vi "Kinesis-basic_program.vi"() -> ()   [LabVIEW 2014]
doc: "André Romero - 2017\nandretec@ifsc.usp.br"
panel:
  out "Numeric 2":i32
  out "GetPOS Y":dbl=10.0
  out "GetPOS X":dbl=10.0 format="%^#1_6e"
  in  "GO Move":bool
  out "Motor 2":bool
  out "Motor 1":bool
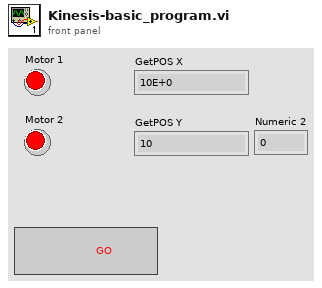
[diagram p1: front panel]
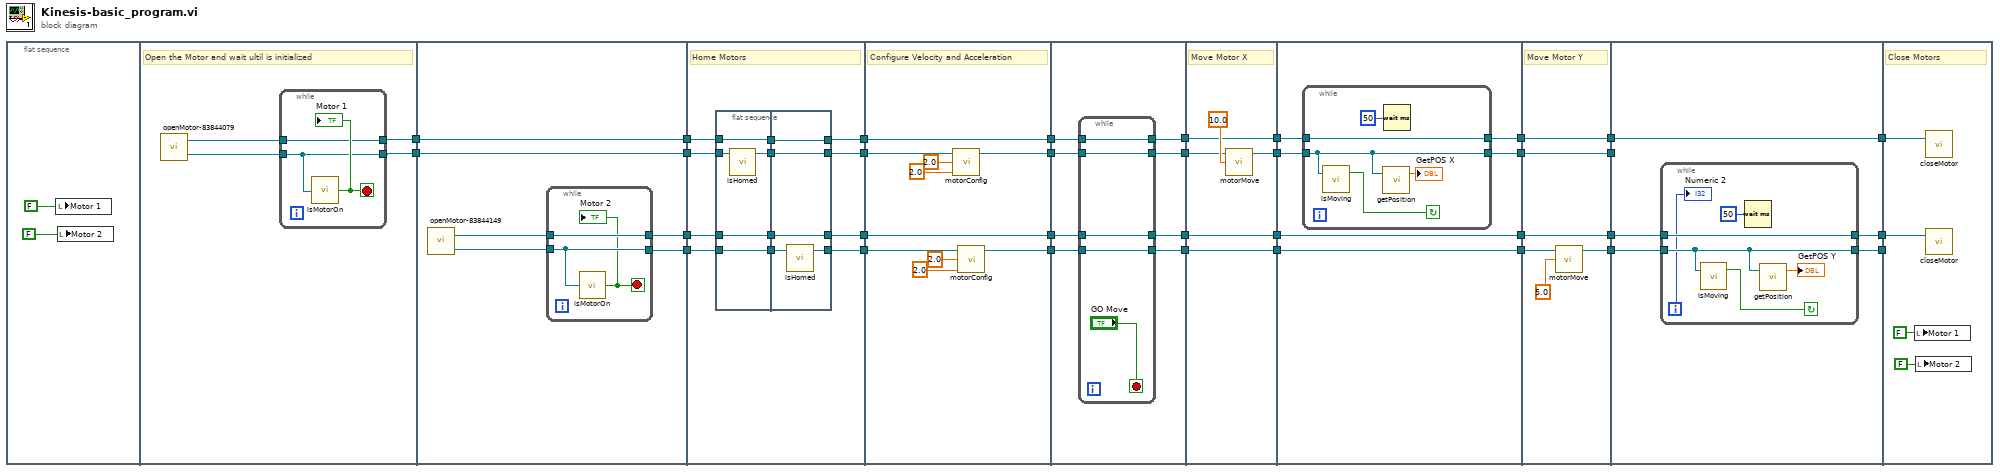
[diagram p0: block diagram]
diagram:
  n1 = flat-sequence {
    tunnel: [w39] -> w10
    tunnel: [w38] -> w8
    tunnel: w10 -> [w48]
    tunnel: [w48] -> w9
    tunnel: w8 -> [w47]
    tunnel: [w47] -> w7
    tunnel: [w46] -> w6
    tunnel: [w45] -> w5
    tunnel: w9 -> [w59]
    tunnel: w7 -> [w58]
    tunnel: [w61] -> w31
    tunnel: w6 -> [w60]
    tunnel: [w62] -> w29
    tunnel: w5 -> [w63]
    tunnel: [w55] -> w33
    tunnel: [w54] -> w27
    tunnel: w33 -> [w82]
    tunnel: [w82] -> w32
    tunnel: w31 -> [w83]
    tunnel: [w83] -> w30
    tunnel: w29 -> [w81]
    tunnel: [w78] -> w28
    tunnel: w27 -> [w74]
    tunnel: [w75] -> w26
    tunnel: w32 -> [w91]
    tunnel: [w90] -> w19
    tunnel: w30 -> [w87]
    tunnel: [w84] -> w22
    tunnel: w28 -> [w85]
    tunnel: [w86] -> w21
    tunnel: w26 -> [w88]
    tunnel: [w89] -> w20
    tunnel: w22 -> [w102]
    tunnel: [w102] -> w18
    tunnel: w21 -> [w97]
    tunnel: [w97] -> w17
    tunnel: w20 -> [w99]
    tunnel: [w98] -> w16
    tunnel: w19 -> [w100]
    tunnel: [w100] -> w15
    tunnel: w18 -> [w104]
    tunnel: [w104] -> w14
    tunnel: w17 -> [w103]
    tunnel: w16 -> [w105]
    tunnel: [w106] -> w13
    tunnel: w15 -> [w108]
    tunnel: [w107] -> w12
    tunnel: [w103] -> w11
    tunnel: w14 -> [w119]
    tunnel: [w119] -> w4
    tunnel: [w114] -> w3
    tunnel: w13 -> [w118]
    tunnel: [w118] -> w2
    tunnel: w12 -> [w117]
    tunnel: [w117] -> w1
    tunnel: w11 -> [w115]
    tunnel: w4 -> [w124]
    tunnel: [w123] -> w25
    tunnel: w3 -> [w120]
    tunnel: [w122] -> w24
    tunnel: w2 -> [_]
    tunnel: w1 -> [w121]
    tunnel: [w121] -> w23
    tunnel: w25 -> [w133]
    tunnel: w24 -> [_]
    tunnel: w23 -> [w134]
    frame #0 {
      n2 = local write "Motor 1"(FALSE ("isConnected")) -> ()
      n3 = local write "Motor 2"(FALSE ("isConnected 2")) -> ()
    }
    frame #1 {
      # "Open the Motor and wait ultil is initialized"
      n4 = call "openMotor-83844079.vi"() -> ("Device"=w37:refnum<k24>, ".NET Refnum out"=w36:refnum<k24>)  [unwired: 2 in]
      n5 = while {
        tunnel: [w41] -> w39
        tunnel: [w40] -> w38
        tunnel: w36 -> [w41]
        tunnel: w37 -> [w40]
        stop <- w42 stop-if-true
        n6 = call "isMotorOn.vi"("Device"=w40) -> ("isConnected"=w42:bool)
        "Motor 1" <- w42
      }
    }
    frame #2 {
      n7 = call "openMotor-83844149.vi"() -> ("Device"=w43:refnum<k24>, ".NET Refnum out"=w44:refnum<k24>)  [unwired: 2 in]
      n8 = while {
        tunnel: w43 -> [w50]
        tunnel: [w51] -> w46
        tunnel: w44 -> [w51]
        tunnel: [w50] -> w45
        stop <- w49 stop-if-true
        n9 = call "isMotorOn.vi"("Device"=w50) -> ("isConnected"=w49:bool)
        "Motor 2" <- w49
      }
    }
    frame #3 {
      # "Home Motors"
      n10 = flat-sequence {
        tunnel: w63 -> [w64]
        tunnel: w60 -> [w68]
        tunnel: w59 -> [w67]
        tunnel: w58 -> [w66]
        tunnel: [w68] -> w57
        tunnel: [w67] -> w56
        tunnel: [w65] -> w53
        tunnel: [w64] -> w52
        tunnel: [w71] -> w54
        tunnel: [w72] -> w55
        tunnel: [w73] -> w61
        tunnel: [w69] -> w62
        tunnel: w57 -> [w73]
        tunnel: w56 -> [w72]
        tunnel: w53 -> [w71]
        tunnel: w52 -> [w70]
        frame #0 {
          n11 = call "isHomed.vi"("Device in"=w66) -> ("Device out"=w65:refnum<k24>)  [unwired: 4 in]
        }
        frame #1 {
          n12 = call "isHomed.vi"("Device in"=w70) -> ("Device out"=w69:refnum<k24>)  [unwired: 4 in]
        }
      }
    }
    frame #4 {
      # "Configure Velocity and Acceleration"
      n13 = call "motorConfig.vi"("Velocity"=2.0 ("MaxVelocity"), "Acceleration"=2.0, "Device in"=w74) -> ("Device out"=w75:refnum<k24>)  [unwired: 2 in]
      n14 = call "motorConfig.vi"("Velocity"=2.0 ("MaxVelocity"), "Acceleration"=2.0, "Device in"=w81) -> ("Device out"=w78:refnum<k24>)  [unwired: 2 in]
    }
    frame #5 {
      n15 = while {
        tunnel: [w95] -> w90
        tunnel: w91 -> [w95]
        tunnel: [w94] -> w89
        tunnel: w88 -> [w94]
        tunnel: w87 -> [w92]
        tunnel: [w93] -> w86
        tunnel: w85 -> [w93]
        tunnel: [w92] -> w84
        stop <- "GO Move" stop-if-true
      }
    }
    frame #6 {
      # "Move Motor X"
      n16 = call "motorMove.vi"("position"=10.0, "Device in"=w99) -> ("Device out"=w98:refnum<k24>)  [unwired: 3 in]
    }
    frame #7 {
      n17 = while {
        tunnel: w108 -> [w113]
        tunnel: w105 -> [w112]
        tunnel: [w113] -> w107
        tunnel: [w112] -> w106
        stop <- w111 continue-if-true
        n18 = call "isMoving.vi"("Device in"=w112) -> ("IsMoving"=w111:bool)  [unwired: 2 in]
        n19 = call "getPosition.vi"("Device"=w112) -> ("GetPOS"=→"GetPOS X":dbl)  [unwired: 2 in]
        n20 = Wait (ms)(milliseconds to wait=u32 50) -> ()  [unwired: 1 out]
      }
    }
    frame #8 {
      # "Move Motor Y"
      n21 = call "motorMove.vi"("position"=5.0, "Device in"=w115) -> ("Device out"=w114:refnum<k24>)  [unwired: 3 in]
    }
    frame #9 {
      n22 = while {
        tunnel: w124 -> [w130]
        tunnel: w120 -> [w129]
        tunnel: [w130] -> w123
        tunnel: [w129] -> w122
        i -> [w125]
        stop <- w128 continue-if-true
        n23 = call "isMoving.vi"("Device in"=w129) -> ("IsMoving"=w128:bool)  [unwired: 2 in]
        n24 = Wait (ms)(milliseconds to wait=u32 50) -> ()  [unwired: 1 out]
        n25 = call "getPosition.vi"("Device"=w129) -> ("GetPOS"=→"GetPOS Y":dbl)  [unwired: 2 in]
        "Numeric 2" <- w125
      }
    }
    frame #10 {
      # "Close Motors"
      n26 = local write "Motor 1"(FALSE ("Motor 1")) -> ()
      n27 = local write "Motor 2"(FALSE ("Motor 2")) -> ()
      n28 = call "closeMotor.vi"(".NET Refnum in"=w134) -> ()  [unwired: 2 in]
      n29 = call "closeMotor.vi"(".NET Refnum in"=w133) -> ()  [unwired: 2 in]
    }
  }
